vi "Read PV-Update.vi"(8 "Error In":errorcluster, 11 "CS++GUIActor in":refnum<class "CS++GUIActor.lvclass">) -> (0 "Error Out":errorcluster, 2 "PV-Update":refnum<user-event>, 3 "CS++GUIActor out":refnum<class "CS++GUIActor.lvclass">)   [LabVIEW 2016, in "CS++GUIActor.lvlib" / "CS++GUIActor.lvclass"]
doc: "Read PV-Update event."
uses:
  CS++GUIActor.lvclass
  Classes/CS++ProcessVariables/ProcessVariable/PV.lvclass
  CS++GUIActor.lvclass/CS++GUIActor.ctl
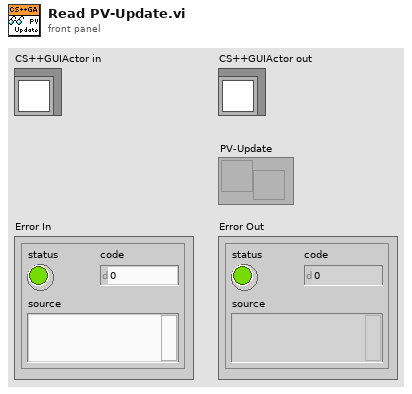
[diagram p1: front panel]
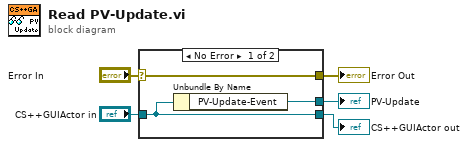
[diagram p0: block diagram]
diagram:
  n1 = case shown="No Error" "Error In" {
    selector: "Error In" -> [w8 w9]
    tunnel: [w8 w9] -> w4
    tunnel: [w7 w10] -> w2
    tunnel: "CS++GUIActor in" -> [w7 w10]
    tunnel: [w6 _] -> w1
    frame No Error {
      n2 = Unbundle By Name(w7) -> ("PV-Update-Event"=w6:refnum<user-event>)
    }
    frame Error {
    }
  }
  "Error Out" <- w4
  "CS++GUIActor out" <- w2
  "PV-Update" <- w1
